vi "failed.vi"() -> ()   [LabVIEW 2014]
uses:
  globalvariables.vi
panel:
  in  "OK Button 2":bool
  in  "OK Button":bool
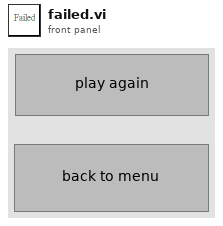
[diagram p1: front panel]
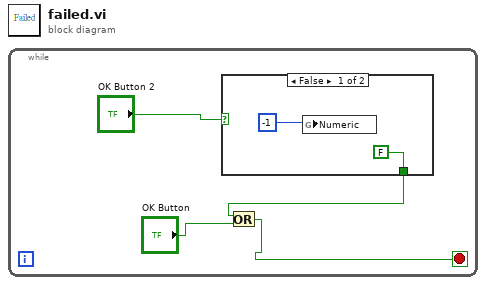
[diagram p0: block diagram]
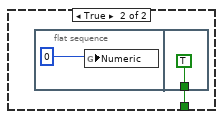
[diagram p2: hidden frame]
diagram:
  n1 = while {
    stop <- w2 stop-if-true
    n2 = case shown="False" "OK Button 2" {
      tunnel: [FALSE w7] -> w1
      frame False {
        n3 = global write "globalvariables.vi" "Numeric"(-1) -> ()
      }
      frame True {
        n4 = flat-sequence {
          tunnel: [TRUE] -> w7
          frame #0 {
            n5 = global write "globalvariables.vi" "Numeric"(0) -> ()
          }
          frame #1 {
          }
        }
      }
    }
    n6 = Or(x=w1, y="OK Button") -> (x .or. y?=w2:bool)
  }
